vi "Test Serialize Args for Windows.vi"() -> (0 "error out":errorcluster)   [LabVIEW 2025]
doc: "Validates that an array of command-line arguments is correctly serialized into a single Windows-compatible argument string. The test ensures that arguments are individually escaped when necessary, correctly quoted, and concatenated in the proper order with spaces between tokens."
uses:
  <vilib>/regexp/Match Regular Expression.xnode
  <vilib>/addons/_JKI Toolkits/Caraya/classes/Test/Test.lvclass
  <vilib>/addons/_JKI Toolkits/Caraya/classes/Assert/Assert.lvclass
  src/Process Executor/Process Executor.lvclass
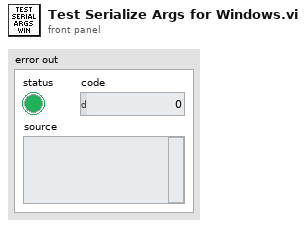
[diagram p1: front panel]
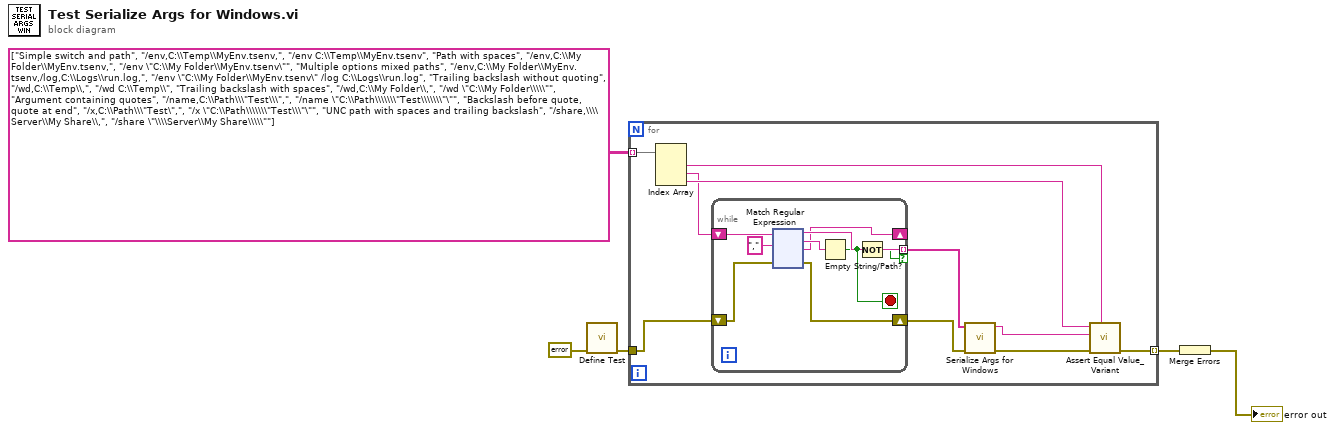
[diagram p0: block diagram]
diagram:
  n1 = call <vilib>:"Define Test.vi"("error in (no error)"=errorcluster {"status"=FALSE, "code"=0, "source"=""}) -> ("error out"=w4:errorcluster)  [unwired: 9 in, 1 out]
  n2 = for {
    tunnel: w4 -> [w7]
    tunnel: string[][] [["Simple switch and path", "/env,C:\\Temp\\MyEnv.tsenv,", "/env C:\\Temp\\MyEnv.tsenv"], ["Path with spaces", "/env,C:\\My Folder\\MyEnv.tsenv,", "/env \"C:\\My Folder\\MyEnv.tsenv\""], ["Multiple options mixed paths", "/env,C:\\My Folder\\MyEnv.tsenv,/log,C:\\Logs\\run.log,", "/env \"C:\\My Folder\\MyEnv.tsenv\" /log C:\\Logs\\run.log"], ["Trailing backslash without quoting", "/wd,C:\\Temp\\,", "/wd C:\\Temp\\"], ["Trailing backslash with spaces", "/wd,C:\\My Folder\\,", "/wd \"C:\\My Folder\\\\\""], ["Argument containing quotes", "/name,C:\\Path\\\"Test\\\",", "/name \"C:\\Path\\\\\\\"Test\\\\\\\"\""], ["Backslash before quote, quote at end", "/x,C:\\Path\\\"Test\",", "/x \"C:\\Path\\\\\\\"Test\\\"\""], ["UNC path with spaces and trailing backslash", "/share,\\\\Server\\My Share\\,", "/share \"\\\\Server\\My Share\\\\\""]] -> [w15] mode=indexing
    tunnel: [w12] -> w1 mode=indexing
    n3 = Index Array(array=w15) -> (element #1=w14:string, element #2=w11:string, element #3=w13:string)  [unwired: 3 in]
    n4 = while {
      tunnel: [w22] -> w9 mode=indexing if=w20
      shift-right: [w18] -> _
      shift-left: w11 -> [w23]
      shift-right: [w16] -> w6
      shift-left: w7 -> [w17]
      stop <- w19 stop-if-true
      n5 = xnode ("Match Regular Expression")("input string"=w23, "regular expression"=",", "error in"=w17) -> ("before match"=w22:string, "whole match"=w21:string, "after match"=w18:string, "error out"=w16:errorcluster)  [unwired: 3 in, 1 out]
      n6 = Empty String/Path?(string/path=w21) -> (empty?=w19:bool)
      n7 = Not(x=w19) -> (.not. x?=w20:bool)
    }
    n8 = call "Serialize Args for Windows.vi"("error in"=w6, "Args"=w9) -> ("error out"=w10:errorcluster, "String"=w8:string)  [unwired: 8 in]
    n9 = call <vilib>:"Assert Equal Value_Variant.vi"("Label"=w14, "error in (no error)"=w10, "Actual"=w8, "Expected"=w13) -> ("error out"=w12:errorcluster)  [unwired: 6 in, 1 out]
  }
  n10 = Merge Errors(w1) -> (→"error out":errorcluster)
